vi "8_Meas_Tdoff.vi"(0 "file path (IN)":path, 1 "VGE":dbl, 2 "VCE":dbl, 5 "Project #":string, 7 "Request #":string, 9 "TEST #":string, 11 "error in (no error)":errorcluster) -> (4 "file path (OUT)":path, 6 "Tdoff (ns)":dbl, 8 "DONE Tdoff":bool, 10 "OFF Region":waveform(dbl)[](graph) caption="Tdoff (ns)", 15 "error out":errorcluster)   [LabVIEW 2020]
uses:
  <vilib>/Waveform/WDTOps.llb/WDT Waveform Duration DBL.vi
  <vilib>/Waveform/WDTOps.llb/WDT Get Waveform Subset DBL.vi
  <vilib>/measure/mascope.llb/Transition Measurements 1 chan.vi
  <vilib>/measure/NI_MAPro.lvlib
panel:
  in  "Decision ?":bool
  out "Cursor a : Channel 3":dbl
  out "Cursor a : Channel 2":dbl
  in  "Cursor a : Channel 3 \nrise edge number":i32=1
  in  "Cursor a : Channel 3 \nrise edge tolerance":dbl=0.1
  in  "Cursor a : Channel 2\nfall edge number":i32=1
  in  "Cursor a : Channel 2\nfall edge tolerance":dbl=0.1
  out "10% Vce":dbl
  out "90% Vge":dbl
  out "measurement info (CH3)":T1 {"ref levels"."ref units" items=["absolute", "relative"]; "ref levels"."high ref level" format="%.2p"; "ref levels"."low ref level" format="%.2p"; "ref levels"."mid ref level" format="%.2p"; "end time" format="%.6e"; "start time" format="%.6e"}
  out "measurement info (CH2)":T1 {"ref levels"."ref units" items=["absolute", "relative"]; "ref levels"."high ref level" format="%.2p"; "ref levels"."low ref level" format="%.2p"; "ref levels"."mid ref level" format="%.2p"; "end time" format="%.6e"; "start time" format="%.6e"}
  in  "reference  levels (CH2 initialize)":T2={"high ref level"=90.0, "mid ref level"=50.0, "low ref level"=10.0, "ref units"=1} {"ref units" items=["absolute", "percent"]; "high ref level" format="%0.2f"; "low ref level" format="%0.2f"; "mid ref level" format="%0.2f"}
  in  "reference  levels (CH3 initialize)":T2={"high ref level"=90.0, "mid ref level"=50.0, "low ref level"=10.0, "ref units"=1} {"ref units" items=["absolute", "percent"]; "high ref level" format="%0.2f"; "low ref level" format="%0.2f"; "mid ref level" format="%0.2f"}
  out "Waveform Graph":waveform(dbl)[](graph)
  # "From 90% Vge to 10% Vce"
  # "Default = 1"
  # "Default = 1"
  # "Default = 0.1"
  # "Default = 0.1"
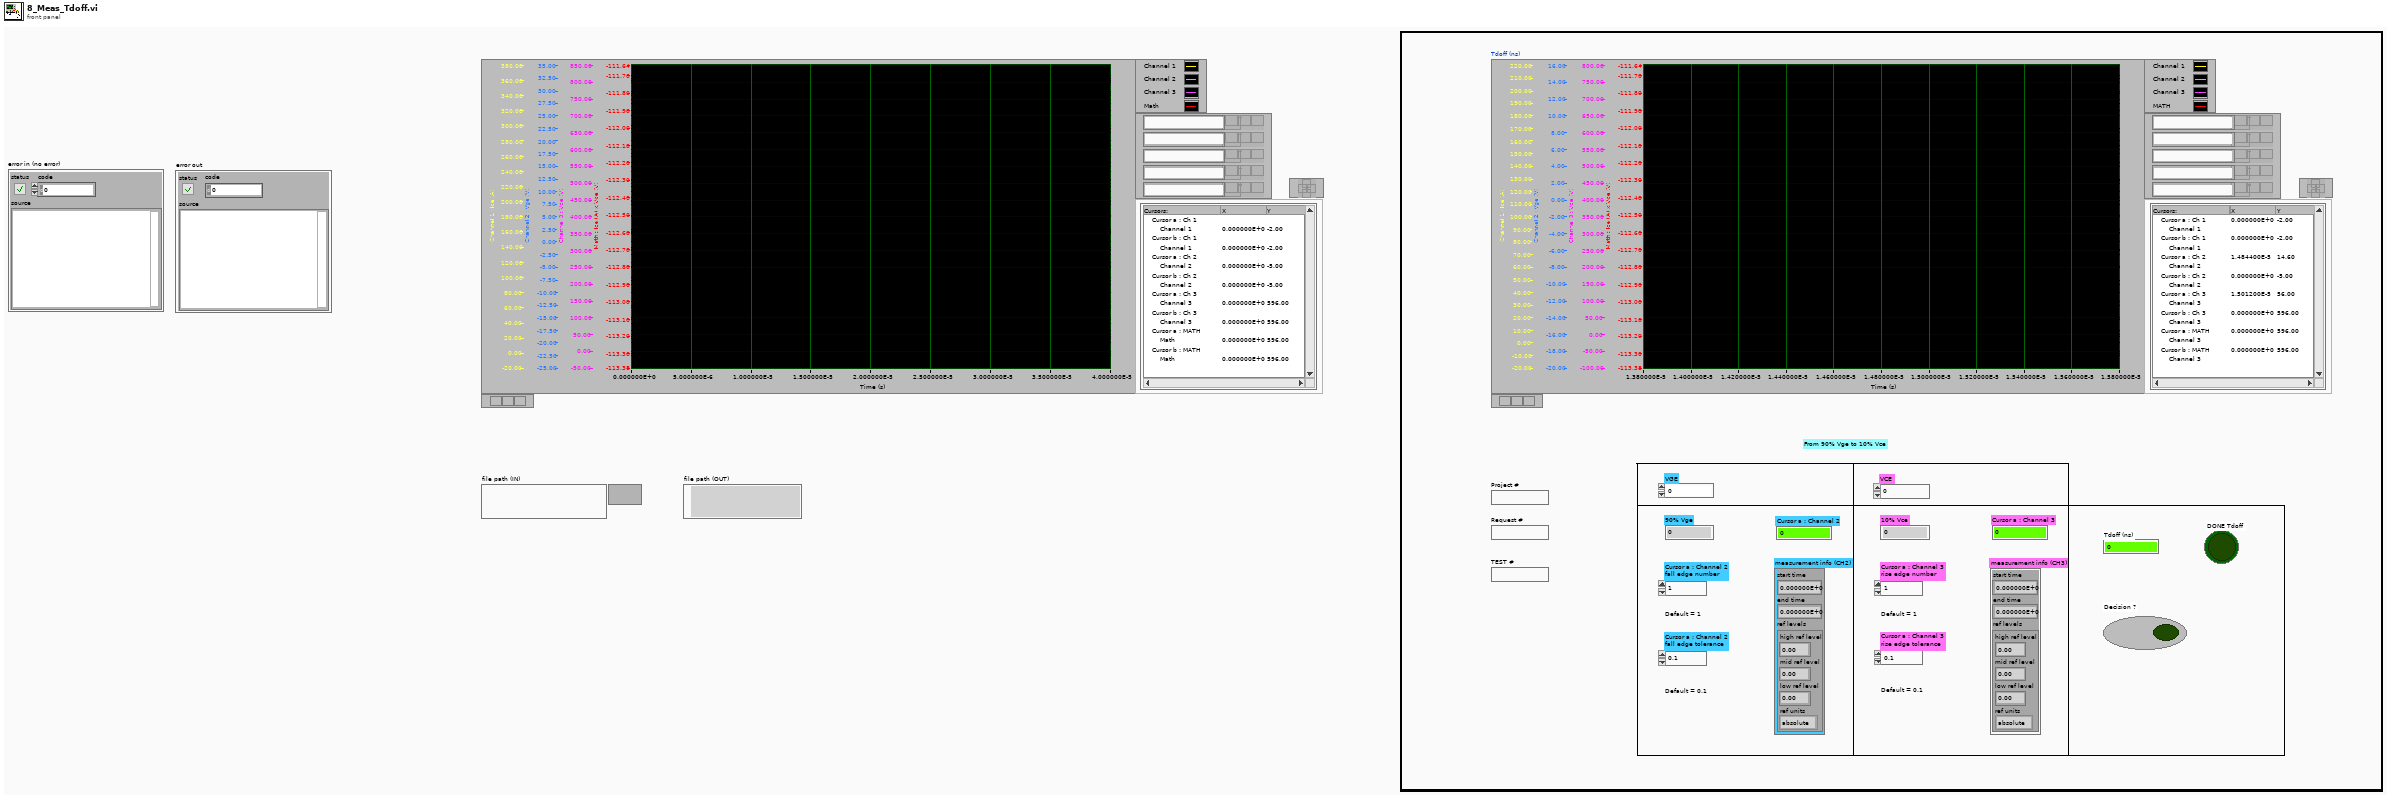
[diagram p1: front panel]
types:
  T1 = cluster{"start time":dbl, "end time":dbl, "ref levels":cluster{"high ref level":dbl, "mid ref level":dbl, "low ref level":dbl, "ref units":u16}}
  T2 = cluster{"high ref level":dbl, "mid ref level":dbl, "low ref level":dbl, "ref units":u16}
  T3 = enum32{"Invalid", "Standard", "Closed", "Hidden", "Minimized", "Maximized"}
  T4 = typedef "imagedata.ctl" = cluster{"image type":i32, "image depth":i32, "image":u8[], "mask":u8[], "colors":u32[], "Rectangle":cluster{"left":i16, "top":i16, "right":i16, "bottom":i16}}
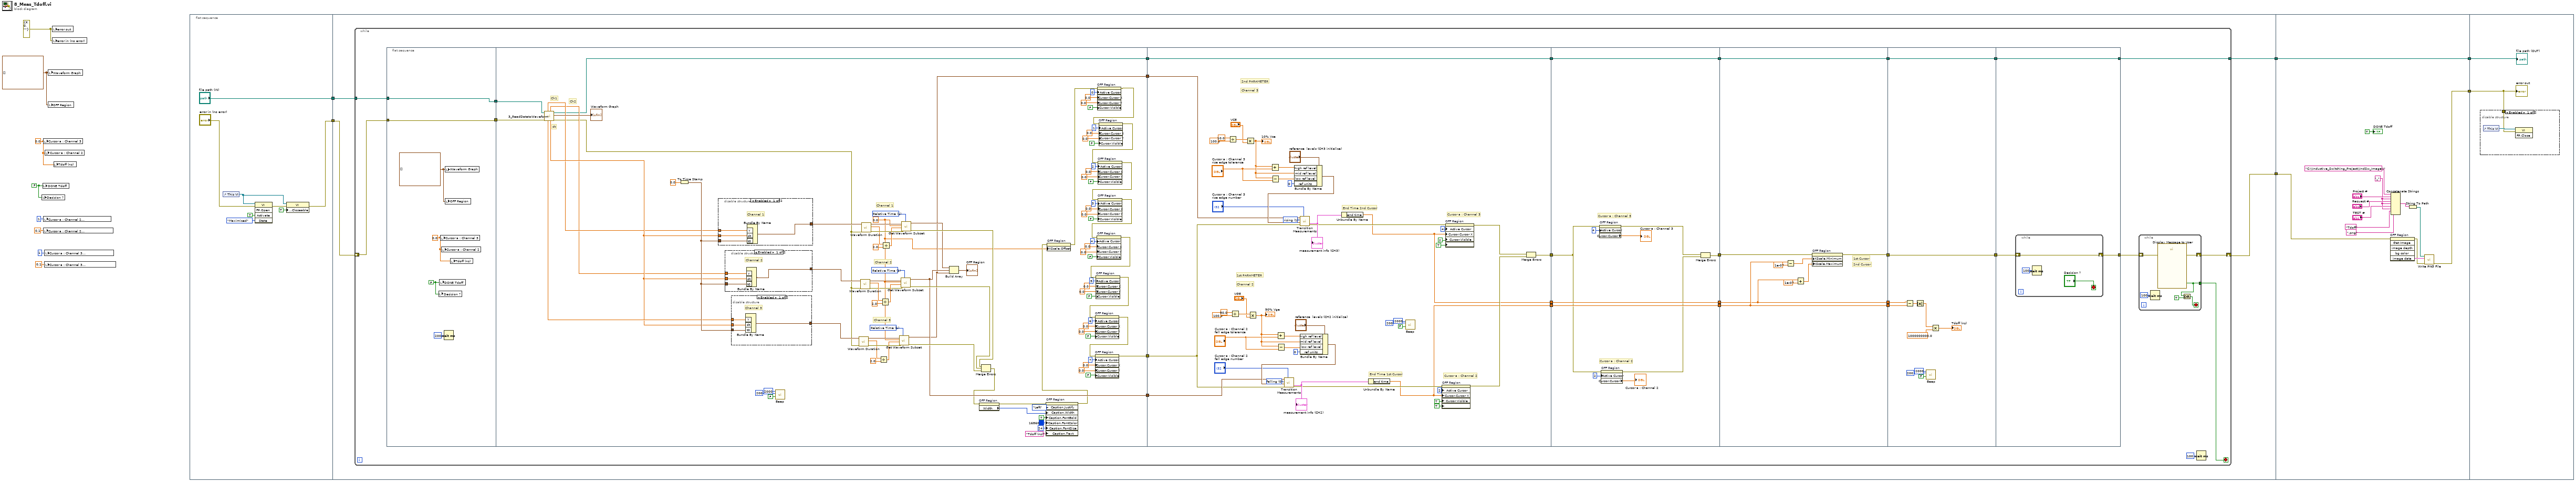
[diagram p0: block diagram]
diagram:
  w12 = 0.0 ("Cursor a : Channel 3")
  w11 = FALSE ("DONE Tdon")
  w13 = waveform(dbl)[] [] ("Waveform Graph")
  w14 = errorcluster {"status"=FALSE, "code"=0, "source"=""} ("error out")
  n1 = local write "Decision ?"(w11) -> ()
  n2 = local write "DONE Tdoff"(w11) -> ()
  n3 = local write "Cursor a : Channel 3"(w12) -> ()
  n4 = local write "Cursor a : Channel 2\nfall edge number"(1 ("Cursor a : Channel 2\nfall edge number")) -> ()
  n5 = local write "Cursor a : Channel 2\nfall edge tolerance"(0.1 ("Cursor a : Channel 2\nfall edge tolerance")) -> ()
  n6 = local write "Cursor a : Channel 3 \nrise edge number"(1 ("Cursor a : Channel 3 \nrise edge number")) -> ()
  n7 = local write "Cursor a : Channel 3 \nrise edge tolerance"(0.1 ("Cursor a : Channel 3 \nrise edge tolerance")) -> ()
  n8 = local write "Cursor a : Channel 2"(w12) -> ()
  n9 = local write "Waveform Graph"(w13) -> ()
  n10 = local write "OFF Region"(w13) -> ()
  n11 = local write "error out"(w14) -> ()
  n12 = local write "error in (no error)"(w14) -> ()
  n13 = local write "Tdoff (ns)"(w12) -> ()
  n14 = flat-sequence {
    tunnel: ["file path (IN)"] -> w10
    tunnel: [w15] -> w5
    tunnel: w10 -> [w26]
    tunnel: [w25] -> w9
    tunnel: [w24] -> w8
    tunnel: w5 -> [w23]
    tunnel: w9 -> [w258]
    tunnel: w8 -> [w257]
    tunnel: [w257] -> w7
    tunnel: [w256] -> w6
    tunnel: w7 -> [w272]
    tunnel: w6 -> [w271]
    frame #0 {
      n15 = control-ref of="This VI"() -> (w20:refnum<vi>)
      n16 = invoke class="VI" method="FP.Open"(reference=w20, error in="error in (no error)", "Activate"=TRUE ("Activate?"), "State"=T3."Maximized") -> (error out=w21:errorcluster)  [unwired: 1 in, 4 out]
      n17 = property class="VI"(reference=w20, error in=w21, "Front Panel.Closeable"=TRUE ("Front Panel Window:Closeable")) -> (error out=w15:errorcluster)  [unwired: 1 out]
    }
    frame #1 {
      n18 = while {
        shift-right: [w31] -> w25
        shift-left: w23 -> [w27]
        tunnel: w26 -> [w29]
        tunnel: [w28] -> w24
        stop <- w32 stop-if-true
        n19 = flat-sequence {
          tunnel: [w54] -> w53
          tunnel: [w55] -> w52
          tunnel: w29 -> [w55]
          tunnel: w27 -> [w54]
          tunnel: w53 -> [w152]
          tunnel: w52 -> [w146]
          tunnel: [w74] -> w51
          tunnel: [w61] -> w50
          tunnel: [w72] -> w49
          tunnel: [w62] -> w48
          tunnel: w51 -> [w188]
          tunnel: w50 -> [w187]
          tunnel: w49 -> [w186]
          tunnel: [w174] -> w47
          tunnel: [w173] -> w46
          tunnel: [w172] -> w45
          tunnel: w48 -> [w171]
          tunnel: [w171] -> w44
          tunnel: w47 -> [w223]
          tunnel: [w223] -> w43
          tunnel: w46 -> [w222]
          tunnel: [w222] -> w42
          tunnel: w45 -> [w216]
          tunnel: [w213] -> w41
          tunnel: w44 -> [w221]
          tunnel: [w221] -> w40
          tunnel: w43 -> [w224]
          tunnel: [w224] -> w39
          tunnel: w42 -> [w225]
          tunnel: [w225] -> w38
          tunnel: w41 -> [w231]
          tunnel: [w230] -> w37
          tunnel: w40 -> [w232]
          tunnel: [w232] -> w36
          tunnel: w39 -> [w242]
          tunnel: w38 -> [w241]
          tunnel: w37 -> [w233]
          tunnel: w36 -> [w236]
          tunnel: [w236] -> w35
          tunnel: [w233] -> w34
          tunnel: w35 -> [w244]
          tunnel: w34 -> [w246]
          tunnel: [w245] -> w33
          tunnel: [w244] -> w28
          frame #0 {
            w58 = 0.0 ("Cursor a : Channel 3")
            w59 = FALSE ("DONE Tdon")
            w57 = waveform(dbl)[] [] ("Waveform Graph")
            n20 = local write "Decision ?"(w59) -> ()
            n21 = local write "DONE Tdoff"(w59) -> ()
            n22 = local write "Cursor a : Channel 3"(w58) -> ()
            n23 = local write "Cursor a : Channel 2"(w58) -> ()
            n24 = Wait (ms)(milliseconds to wait=u32 200) -> ()  [unwired: 1 out]
            n25 = local write "Waveform Graph"(w57) -> ()
            n26 = local write "OFF Region"(w57) -> ()
            n27 = local write "Tdoff (ns)"(w58) -> ()
          }
          frame #1 {
            w60 = 0.0 ("start samples/time")
            w127 = u16 1 items=["Samples", "Relative Time"] ("start/duration format")
            w138 = u16 1 items=["Samples", "Relative Time"] ("start/duration format")
            w139 = u16 1 items=["Samples", "Relative Time"] ("start/duration format")
            # "Channel 1"
            # "Channel 3"
            # "Channel 2"
            # "dt"
            # "Ch2"
            # "Ch1"
            n28 = call "3_ReadDatatoWaveform.vi"("error in (no error)"=w152, "file path (IN)"=w146) -> ("error out"=w121:errorcluster, "Waveform Graph"=→"Waveform Graph":waveform(dbl)[], "file path (OUT)"=w62:path, "dt"=w147:dbl, "Ch 2 Data"=w144:dbl[], "Ch 3 Data"=w148:dbl[], "Ch 1 Data"=w145:dbl[])  [unwired: 3 in]
            n29 = To Time Stamp(1:0.0 ("number")) -> (0:w149:timestamp)
            n30 = disable-structure shown="Enabled" {
              disable-tunnel: w149 -> [w156 _]
              disable-tunnel: w147 -> [w155 _]
              disable-tunnel: w145 -> [w154 _]
              disable-tunnel: [w153 _] -> w126
              frame Enabled {
                # "Channel 1"
                n31 = Bundle By Name("Y"=w154, "dt"=w155, "t0"=w156) -> (w153:waveform(dbl))  [unwired: 1 in]
              }
              frame Disabled {
              }
            }
            n32 = disable-structure shown="Enabled" {
              disable-tunnel: w149 -> [w160 _]
              disable-tunnel: w147 -> [w159 _]
              disable-tunnel: w144 -> [w158 _]
              disable-tunnel: [w157 _] -> w125
              frame Enabled {
                # "Channel 2"
                n33 = Bundle By Name("Y"=w158, "dt"=w159, "t0"=w160) -> (w157:waveform(dbl))  [unwired: 1 in]
              }
              frame Disabled {
              }
            }
            n34 = disable-structure shown="Enabled" {
              disable-tunnel: w149 -> [w164 _]
              disable-tunnel: w147 -> [w163 _]
              disable-tunnel: w148 -> [w162 _]
              disable-tunnel: [w161 _] -> w124
              frame Enabled {
                # "Channel 3"
                n35 = Bundle By Name("Y"=w162, "dt"=w163, "t0"=w164) -> (w161:waveform(dbl))  [unwired: 1 in]
              }
              frame Disabled {
              }
            }
            n36 = call <vilib>:"Beep.vi"("use system alert? (T)"=FALSE, "duration (msec)"=u32 200, "frequency (Hz)"=u32 2000) -> ()  [unwired: 9 in]
            n37 = call-poly <vilib>:"Waveform Duration.vi"("error in (no error)"=w121, "waveform in"=w124) -> ("error out"=w132:errorcluster, "duration"=w129:dbl, "waveform out"=w131:waveform(dbl))  [unwired: 7 in]
            n38 = call-poly <vilib>:"Waveform Duration.vi"("error in (no error)"=w121, "waveform in"=w125) -> ("error out"=w133:errorcluster, "duration"=w136:dbl, "waveform out"=w134:waveform(dbl))  [unwired: 7 in]
            n39 = call-poly <vilib>:"Waveform Duration.vi"("error in (no error)"=w121, "waveform in"=w126) -> ("error out"=w143:errorcluster, "duration"=w140:dbl, "waveform out"=w142:waveform(dbl))  [unwired: 7 in]
            n40 = Divide(x=w129, y=2.0) -> (x/y=w128:dbl)
            n41 = Divide(x=w136, y=2.0) -> (x/y=w137:dbl)
            n42 = Divide(x=w140, y=2.0) -> (x/y=w122:dbl)
            n43 = call-poly <vilib>:"Get Waveform Subset.vi"("start/duration format"=w127, "error in (no error)"=w132, "duration"=w128, "start samples/time"=w60, "waveform in"=w131) -> ("error out"=w118:errorcluster, "waveform out"=w61:waveform(dbl))  [unwired: 1 in, 2 out]
            n44 = call-poly <vilib>:"Get Waveform Subset.vi"("start/duration format"=w138, "error in (no error)"=w133, "duration"=w137, "start samples/time"=w60, "waveform in"=w134) -> ("error out"=w119:errorcluster, "waveform out"=w74:waveform(dbl))  [unwired: 1 in, 2 out]
            n45 = call-poly <vilib>:"Get Waveform Subset.vi"("start/duration format"=w139, "error in (no error)"=w143, "duration"=w122, "start samples/time"=w60, "waveform in"=w142) -> ("error out"=w120:errorcluster, "waveform out"=w73:waveform(dbl))  [unwired: 1 in, 2 out]
            n46 = Build Array(w73, w74, w61) -> (→"OFF Region":waveform(dbl)[])
            n47 = Merge Errors(w120, w119, w118) -> (w70:errorcluster)
            n48 = property on="OFF Region" class="WFGraph (strict)"(error in=w70) -> (error out=w69:errorcluster, "Width"=w68:u32)  [unwired: 1 in, 1 out]
            n49 = property on="OFF Region" class="WFGraph (strict)"(error in=w69, "Caption.Justify"=enum16{"Left", "Center", "Right"}."Left" ("Caption.Justification"), "Caption.Width"=w68, "Caption.FontBold"=TRUE ("Caption.Font:Bold"), "Caption.FontColor"=u32 16860 ("Caption.Font:Color"), "Caption.FontSize"=u32 24 ("Caption.Font:Size"), "Caption.Text"="Tdoff (ns)") -> (error out=w64:errorcluster)  [unwired: 1 in, 1 out]
            n50 = property on="OFF Region" class="WFGraph (strict)"(error in=w64, "XScale.Offset"=w60) -> (error out=w98:errorcluster)  [unwired: 1 in, 1 out]
            n51 = property on="OFF Region" class="WFGraph (strict)"(error in=w98, "Active Cursor"=u32 0, "Cursor.Cursor X"=0.0 ("Cursor.Cursor Position:Cursor X"), "Cursor.Cursor Y"=0.0 ("Cursor.Cursor Position:Cursor Y"), "Cursor.Visible"=FALSE) -> (error out=w97:errorcluster)  [unwired: 1 in, 1 out]
            n52 = property on="OFF Region" class="WFGraph (strict)"(error in=w97, "Active Cursor"=u32 1, "Cursor.Cursor X"=0.0 ("Cursor.Cursor Position:Cursor X"), "Cursor.Cursor Y"=0.0 ("Cursor.Cursor Position:Cursor Y"), "Cursor.Visible"=FALSE) -> (error out=w96:errorcluster)  [unwired: 1 in, 1 out]
            n53 = property on="OFF Region" class="WFGraph (strict)"(error in=w96, "Active Cursor"=u32 2, "Cursor.Cursor X"=0.0 ("Cursor.Cursor Position:Cursor X"), "Cursor.Cursor Y"=0.0 ("Cursor.Cursor Position:Cursor Y"), "Cursor.Visible"=FALSE) -> (error out=w95:errorcluster)  [unwired: 1 in, 1 out]
            n54 = property on="OFF Region" class="WFGraph (strict)"(error in=w95, "Active Cursor"=u32 3, "Cursor.Cursor X"=0.0 ("Cursor.Cursor Position:Cursor X"), "Cursor.Cursor Y"=0.0 ("Cursor.Cursor Position:Cursor Y"), "Cursor.Visible"=FALSE) -> (error out=w78:errorcluster)  [unwired: 1 in, 1 out]
            n55 = property on="OFF Region" class="WFGraph (strict)"(error in=w78, "Active Cursor"=u32 4, "Cursor.Cursor X"=0.0 ("Cursor.Cursor Position:Cursor X"), "Cursor.Cursor Y"=0.0 ("Cursor.Cursor Position:Cursor Y"), "Cursor.Visible"=FALSE) -> (error out=w77:errorcluster)  [unwired: 1 in, 1 out]
            n56 = property on="OFF Region" class="WFGraph (strict)"(error in=w77, "Active Cursor"=u32 5, "Cursor.Cursor X"=0.0 ("Cursor.Cursor Position:Cursor X"), "Cursor.Cursor Y"=0.0 ("Cursor.Cursor Position:Cursor Y"), "Cursor.Visible"=FALSE) -> (error out=w76:errorcluster)  [unwired: 1 in, 1 out]
            n57 = property on="OFF Region" class="WFGraph (strict)"(error in=w76, "Active Cursor"=u32 6, "Cursor.Cursor X"=0.0 ("Cursor.Cursor Position:Cursor X"), "Cursor.Cursor Y"=0.0 ("Cursor.Cursor Position:Cursor Y"), "Cursor.Visible"=FALSE) -> (error out=w75:errorcluster)  [unwired: 1 in, 1 out]
            n58 = property on="OFF Region" class="WFGraph (strict)"(error in=w75, "Active Cursor"=u32 7, "Cursor.Cursor X"=0.0 ("Cursor.Cursor Position:Cursor X"), "Cursor.Cursor Y"=0.0 ("Cursor.Cursor Position:Cursor Y"), "Cursor.Visible"=FALSE) -> (error out=w72:errorcluster)  [unwired: 1 in, 1 out]
          }
          frame #2 {
            w203 = u16 0 items=["falling", "rising"] ("polarity (rising)")
            w204 = u16 1 items=["falling", "rising"] ("polarity (rising)")
            # "Cursor a : Channel 2"
            # "Cursor a : Channel 3"
            # "End Time 2nd Cursor"
            # "End Time 1st Cursor"
            # "2nd PARAMETER"
            # "Channel 3"
            # "1st PARAMETER"
            # "Channel 2"
            n59 = Divide(x=10.0, y=100.0) -> (x/y=w212:dbl)
            n60 = Divide(x=90.0, y=100.0) -> (x/y=w208:dbl)
            n61 = Multiply(x=w212, y="VCE") -> (x*y=w189:dbl)
            "10% Vce" <- w189
            n62 = Multiply(x=w208, y="VGE") -> (x*y=w196:dbl)
            "90% Vge" <- w196
            n63 = Add(x=w189, y="Cursor a : Channel 3 \nrise edge tolerance") -> (x+y=w195:dbl)
            n64 = Subtract(x=w189, y="Cursor a : Channel 3 \nrise edge tolerance") -> (x-y=w194:dbl)
            n65 = Add(x=w196, y="Cursor a : Channel 2\nfall edge tolerance") -> (x+y=w202:dbl)
            n66 = Subtract(x=w196, y="Cursor a : Channel 2\nfall edge tolerance") -> (x-y=w201:dbl)
            n67 = Bundle By Name(cluster="reference  levels (CH3 initialize)", "high ref level"=w195, "mid ref level"=w189, "low ref level"=w194, "ref units"=u16 0) -> (w191:T2)
            n68 = call-poly <vilib>:"Transition Measurements.vi"("edge number (1)"="Cursor a : Channel 3 \nrise edge number", "error in (no error)"=w186, "reference levels"=w191, "polarity (rising)"=w204, "signal in"=w187) -> ("error out"=w183:errorcluster, "measurement info"=w190:T1)  [unwired: 1 in, 4 out]
            "measurement info (CH3)" <- w190
            n69 = Bundle By Name(cluster="reference  levels (CH2 initialize)", "high ref level"=w202, "mid ref level"=w196, "low ref level"=w201, "ref units"=u16 0) -> (w198:T2)
            n70 = call-poly <vilib>:"Transition Measurements.vi"("edge number (1)"="Cursor a : Channel 2\nfall edge number", "error in (no error)"=w186, "reference levels"=w198, "polarity (rising)"=w203, "signal in"=w188) -> ("error out"=w180:errorcluster, "measurement info"=w197:T1)  [unwired: 1 in, 4 out]
            "measurement info (CH2)" <- w197
            n71 = Unbundle By Name(w190) -> ("end time"=w174:dbl)
            n72 = Unbundle By Name(w197) -> ("end time"=w173:dbl)
            n73 = call <vilib>:"Beep.vi"("use system alert? (T)"=FALSE, "duration (msec)"=u32 200, "frequency (Hz)"=u32 2000) -> ()  [unwired: 9 in]
            n74 = property on="OFF Region" class="WFGraph (strict)"(error in=w180, "Active Cursor"=u32 2, "Cursor.Cursor X"=w173, "Cursor.Visible"=TRUE, "Cursor.Cursor Name Visible"=TRUE) -> (error out=w175:errorcluster)  [unwired: 1 in, 1 out]
            n75 = property on="OFF Region" class="WFGraph (strict)"(error in=w183, "Active Cursor"=u32 4, "Cursor.Cursor X"=w174, "Cursor.Visible"=TRUE, "Cursor.Cursor Name Visible"=TRUE) -> (error out=w176:errorcluster)  [unwired: 1 in, 1 out]
            n76 = Merge Errors(w176, w175) -> (w172:errorcluster)
          }
          frame #3 {
            # "Cursor a : Channel 3"
            # "Cursor a : Channel 2"
            n77 = property on="OFF Region" class="WFGraph (strict)"(error in=w216, "Active Cursor"=u32 4) -> (error out=w215:errorcluster, "Cursor.Cursor Y"=→"Cursor a : Channel 3":dbl)  [unwired: 1 in, 1 out]
            n78 = property on="OFF Region" class="WFGraph (strict)"(error in=w216, "Active Cursor"=u32 2) -> (error out=w214:errorcluster, "Cursor.Cursor Y"=→"Cursor a : Channel 2":dbl)  [unwired: 1 in, 1 out]
            n79 = Merge Errors(w215, w214) -> (w213:errorcluster)
          }
          frame #4 {
            # "2nd Cursor"
            # "1st Cursor"
            n80 = Subtract(x=w225, y=1e-07) -> (x-y=w226:dbl)
            n81 = Add(x=w224, y=1e-07) -> (x+y=w227:dbl)
            n82 = property on="OFF Region" class="WFGraph (strict)"(error in=w231, "XScale.Minimum"=w226, "XScale.Maximum"=w227) -> (error out=w230:errorcluster)  [unwired: 1 in, 1 out]
          }
          frame #5 {
            n83 = Subtract(x=w242, y=w241) -> (x-y=w235:dbl)
            n84 = Absolute Value(x=w235) -> (abs(x)=w234:dbl)
            n85 = call <vilib>:"Beep.vi"("use system alert? (T)"=FALSE, "duration (msec)"=u32 200, "frequency (Hz)"=u32 2000) -> ()  [unwired: 9 in]
            n86 = Multiply(x=w234, y=1000000000.0) -> (x*y=→"Tdoff (ns)":dbl)
          }
          frame #6 {
            n87 = while {
              shift-right: [w247] -> w245
              shift-left: w246 -> [w247]
              stop <- "Decision ?" stop-if-true
              n88 = Wait (ms)(milliseconds to wait=u32 100) -> ()  [unwired: 1 out]
            }
          }
        }
        n89 = while {
          tunnel: [w251] -> w32
          shift-right: [w254] -> w31
          shift-left: w33 -> [w255]
          stop <- w253 stop-if-true
          n90 = Wait (ms)(milliseconds to wait=u32 100) -> ()  [unwired: 1 out]
          n91 = call "Display Message to User"("error in (no error)"=w255) -> ("error out"=w254:errorcluster, "NO"=w251:bool)  [unwired: 9 in]
          n92 = Or(x=w251, y=TRUE) -> (x .or. y?=w253:bool)
        }
        n93 = Wait (ms)(milliseconds to wait=u32 100) -> ()  [unwired: 1 out]
      }
    }
    frame #2 {
      w262 = "_"
      n94 = invoke on="OFF Region" class="WFGraph (strict)" method="Get Image"(error in=w258) -> (error out=w264:errorcluster, "image data"=w267:T4)  [unwired: 5 in, 4 out]
      n95 = Concatenate Strings("C:\\Inductive_Switching_Project\\IndSw_Image\\" ("string"), "Project #", w262, "Request #", w262, "TEST #", w262, "Tdoff" ("string"), ".png" ("string")) -> (w268:string)
      n96 = String To Path(string=w268) -> (path=w266:path)
      n97 = call <vilib>:"Write PNG File.vi"("error in (no error)"=w264, "image data"=w267, "path to PNG file"=w266) -> ("error out"=w256:errorcluster)  [unwired: 7 in, 1 out]
      "DONE Tdoff" <- TRUE ("DONE Tdon")
    }
    frame #3 {
      n98 = disable-structure shown="Enabled" {
        disable-tunnel: w271 -> [w273 _]
        frame Enabled {
          n99 = control-ref of="This VI"() -> (w274:refnum<vi>)
          n100 = invoke class="VI" method="FP.Close"(reference=w274, error in=w273) -> ()  [unwired: 1 in, 3 out]
        }
        frame Disabled {
        }
      }
      "error out" <- w271
      "file path (OUT)" <- w272
    }
  }
